vi "Pendulum Reset.vi"(11 "instance":i32) -> (3 "function return":i32)   [LabVIEW 2025, in "pendulumApp.lvlib"]
doc: "OOTB_API int Pendulum_Reset(int instance,double retry_mS);\n\nOOTB_API int Pendulum_Reset(int instance);"
uses:
  pendulumApp.lvlib
  pendulumApp.dll
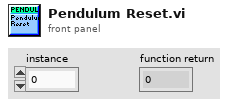
[diagram p1: front panel]
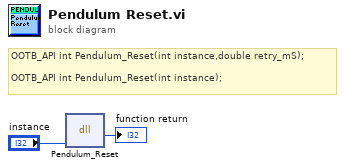
[diagram p0: block diagram]
diagram:
  # "OOTB_API\tint Pendulum_Reset(int instance,double retry_mS);\n\nOOTB_API\tint Pendulum_Reset(int instance);"
  n1 = dll-call lib="C:/Users/noaht/School/Fall 2025/Controls Lab/Lab 4/FA25_pend_Lab3_4/SADI_Pendulum_lib/pendulumApp.*" fn="Pendulum_Reset"("instance"="instance") -> (→"function return":i32)  [unwired: 4 in, 2 out]
